vi "Example Main Host.vi"() -> ()   [LabVIEW 2018]
uses:
  <vilib>/Utility/Variable/NI_VariableUtilities.lvlib
panel:
  in  "Stop":bool
  out "Force (N)":cluster{"Double":dbl, "Double":dbl}(graph)
  out "Iteration Duration (us)":i32
  out "Encoder Angle (deg)":cluster{"Double":dbl, "Double":dbl}(graph)
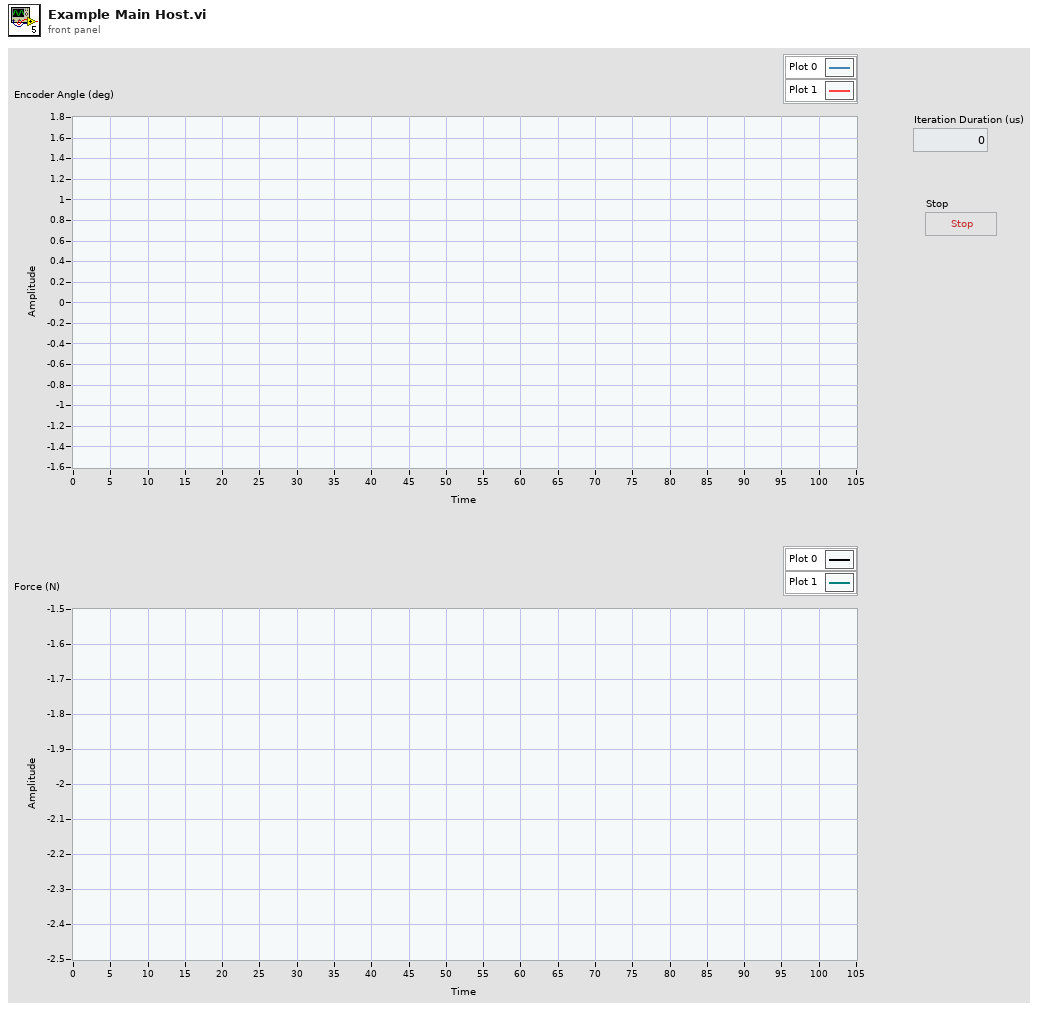
[diagram p1: front panel]
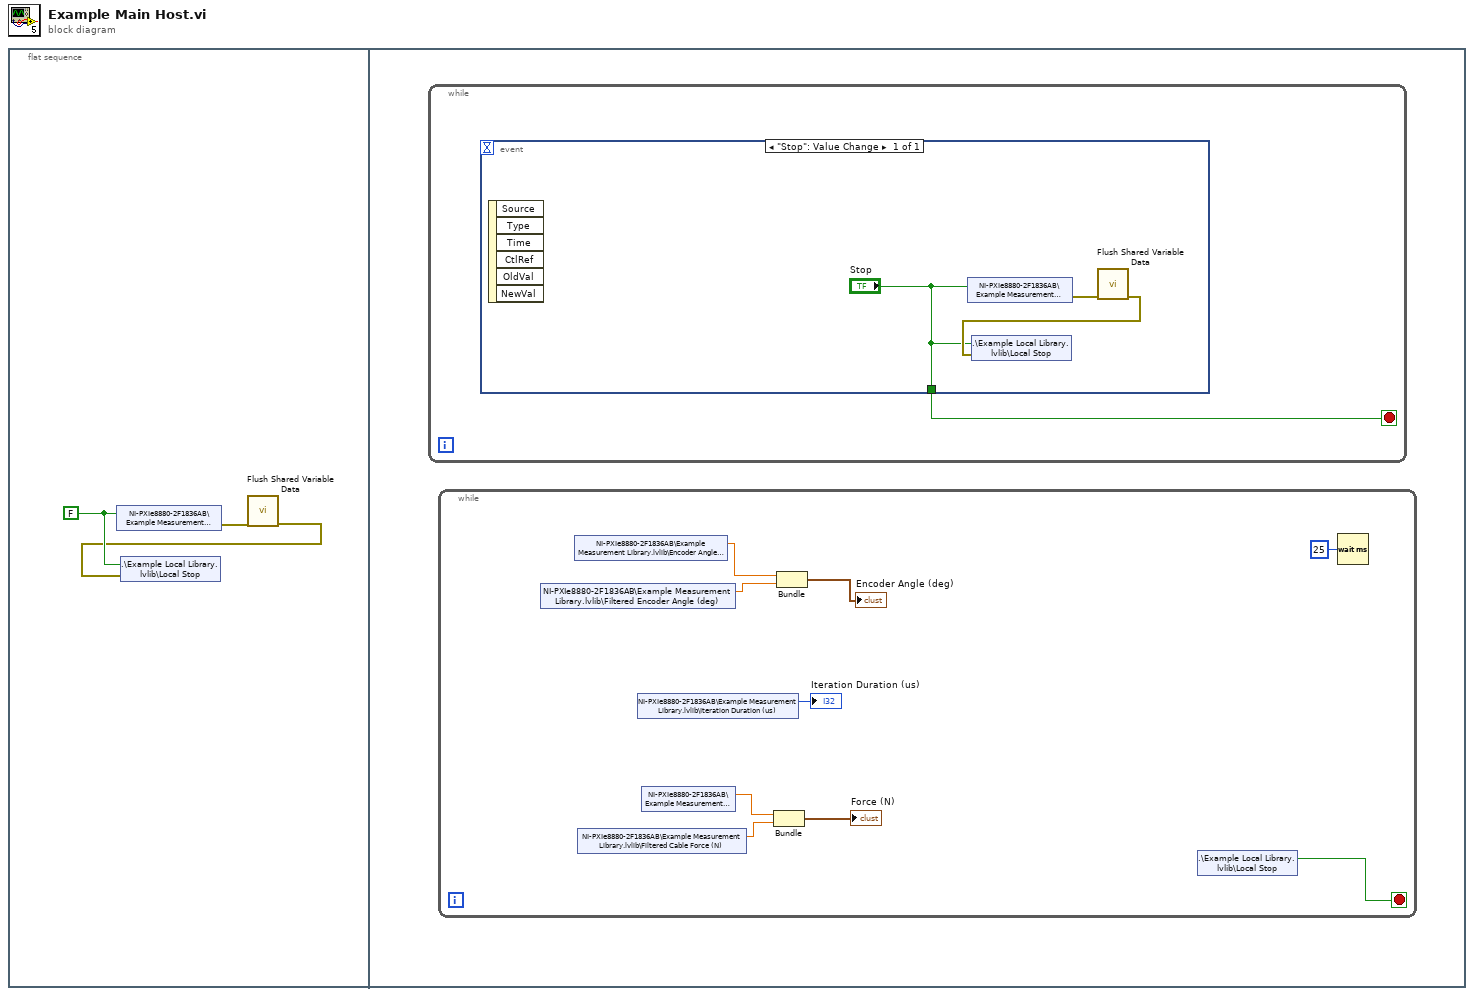
[diagram p0: block diagram]
diagram:
  n1 = flat-sequence {
    frame #0 {
      w3 = FALSE ("Target Stop")
      n2 = shared-variable "NI-PXIe8880-2F1836AB\\Example Measurement Library.lvlib\\Target Stop"(w3) -> (error out=w2:errorcluster)  [unwired: 1 in]
      n3 = call <vilib>:"Flush Shared Variable Data.vi"("error in (no error)"=w2) -> ("error out"=w1:errorcluster)  [unwired: 10 in]
      n4 = shared-variable ".\\Example Local Library.lvlib\\Local Stop"(w3, error in=w1) -> ()  [unwired: 1 out]
    }
    frame #1 {
      n5 = while {
        stop <- w4 stop-if-true
        n6 = event shown="[0] \"Stop\": Value Change" {
          selector: _ -> [_]
          dyn-events: _ -> [_]
          timeout: _ -> [_]
          tunnel: ["Stop"] -> w4
          event "Stop": Value Change {
            n7 = event-data() -> ()  [unwired: 1 in, 6 out]
            n8 = shared-variable "NI-PXIe8880-2F1836AB\\Example Measurement Library.lvlib\\Target Stop"("Stop") -> (error out=w7:errorcluster)  [unwired: 1 in]
            n9 = call <vilib>:"Flush Shared Variable Data.vi"("error in (no error)"=w7) -> ("error out"=w6:errorcluster)  [unwired: 10 in]
            n10 = shared-variable ".\\Example Local Library.lvlib\\Local Stop"("Stop", error in=w6) -> ()  [unwired: 1 out]
          }
        }
      }
      n11 = while {
        stop <- w8 stop-if-true
        n12 = shared-variable "NI-PXIe8880-2F1836AB\\Example Measurement Library.lvlib\\Filtered Encoder Angle (deg)"() -> (w9:dbl)  [unwired: 1 in, 1 out]
        n13 = shared-variable "NI-PXIe8880-2F1836AB\\Example Measurement Library.lvlib\\Encoder Angle (deg)"() -> (w10:dbl)  [unwired: 1 in, 1 out]
        n14 = shared-variable "NI-PXIe8880-2F1836AB\\Example Measurement Library.lvlib\\Filtered Cable Force (N)"() -> (w13:dbl)  [unwired: 1 in, 1 out]
        n15 = shared-variable "NI-PXIe8880-2F1836AB\\Example Measurement Library.lvlib\\Iteration Duration (us)"() -> (→"Iteration Duration (us)":i32)  [unwired: 1 in, 1 out]
        n16 = shared-variable "NI-PXIe8880-2F1836AB\\Example Measurement Library.lvlib\\Force (N)"() -> (w14:dbl)  [unwired: 1 in, 1 out]
        n17 = Bundle("Double"=w14, "Double"=w13) -> (→"Force (N)":cluster{"Double":dbl, "Double":dbl})  [unwired: 1 in]
        n18 = Bundle("Double"=w10, "Double"=w9) -> (→"Encoder Angle (deg)":cluster{"Double":dbl, "Double":dbl})  [unwired: 1 in]
        n19 = shared-variable ".\\Example Local Library.lvlib\\Local Stop"() -> (w8:bool)  [unwired: 1 in, 1 out]
        n20 = Wait (ms)(milliseconds to wait=u32 25) -> ()  [unwired: 1 out]
      }
    }
  }
